vi "Read Process.vi"(8 "error in (no error)":errorcluster, 11 "Process Test in":refnum<class "Process Dev Test.lvclass">) -> (0 "error out":errorcluster, 2 "Process.lvclass":refnum<class "Process.lvclass">, 3 "Process Test out":refnum<class "Process Dev Test.lvclass">)   [LabVIEW 2020, in "Process Dev Test.lvclass"]
uses:
  Process Dev Test.lvclass
  source/Framework/Process/Process.lvclass
  C:/Git/astemes-triarc-framework/source/Framework Test/Base Class Test/Base Test.lvclass
  source/Framework Test Suite/Base Class Test/Base Test.lvclass/Base Test.ctl
  source/Framework/Base/Base.lvclass
  Process Dev Test.lvclass/Process Dev Test.ctl
  source/Framework Test Suite/Base Class Test/Base Test.lvclass
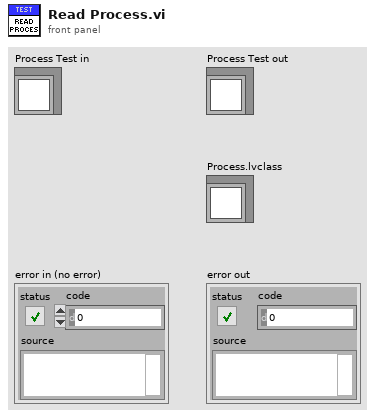
[diagram p1: front panel]
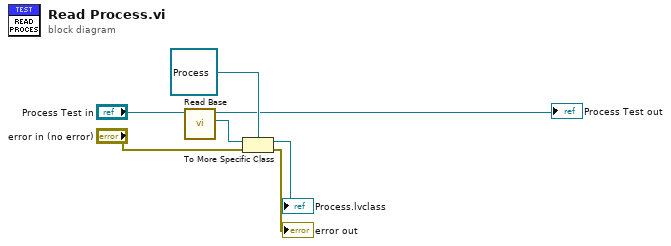
[diagram p0: block diagram]
diagram:
  n1 = call "Read Base.vi"("Base Class Test In"="Process Test in") -> ("Base.lvclass"=w4:refnum<class "Base.lvclass">, "Base Class Test Out"=→"Process Test out":refnum<class "Process Dev Test.lvclass">)  [unwired: 8 in, 1 out]
  n2 = To More Specific Class(target class=refnum<class "Process.lvclass"> refnum ("Process.lvclass"), reference=w4, error in="error in (no error)") -> (specific class reference=→"Process.lvclass":refnum<class "Process.lvclass">, error out=→"error out":errorcluster)
